vi "Initialize.vi"(8 "error in":errorcluster, 9 "Application Directory":path, 10 "Device":string, 11 "Oscilloscope in":refnum<class "Oscilloscope.lvclass">) -> (0 "error out":errorcluster, 3 "Oscilloscope out":refnum<class "Oscilloscope.lvclass">)   [LabVIEW 2019, in "Oscilloscope.lvlib" / "Oscilloscope.lvclass"]
uses:
  Oscilloscope.lvclass
  builds/Instruments/Instruments.lvlibp/Library/Instruments.lvclass
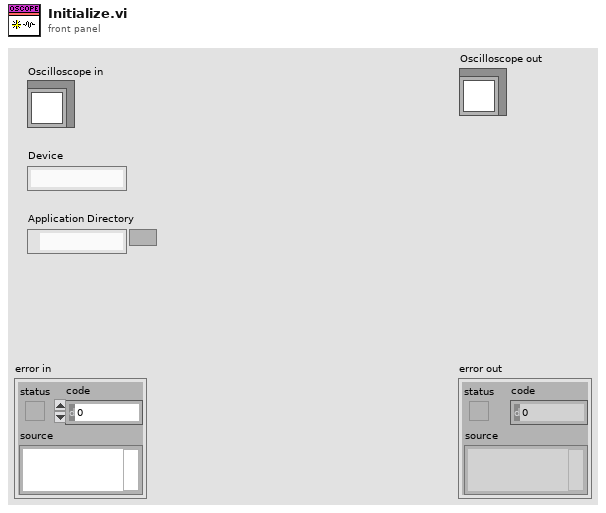
[diagram p1: front panel]
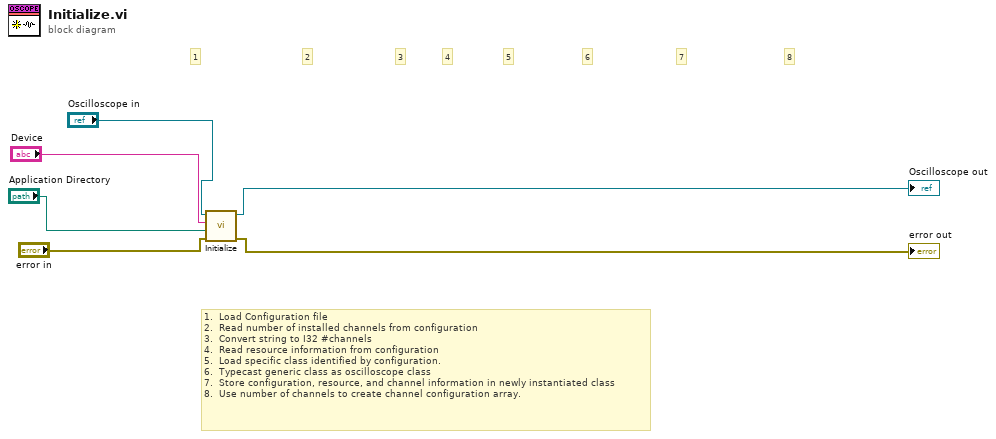
[diagram p0: block diagram]
diagram:
  # "1.  Load Configuration file\n2.  Read number of installed channels from configuration\n3.  Convert string to I32 #channels\n4.  Read resource information from configuration\n5.  Load specific class identified by configuration.\n6.  Typecast generic class as oscilloscope class\n7.  Store configuration, resource, and channel information in newly instantiated class\n8.  Use number of channels to create channel configuration array."
  # "8"
  # "7"
  # "6"
  # "5"
  # "4"
  # "3"
  # "2"
  # "1"
  n1 = call-parent "Initialize.vi"("error in"="error in", "Path"="Application Directory", "Device"="Device", "Instruments in"="Oscilloscope in") -> ("error out"=→"error out":errorcluster, "Instruments out"=→"Oscilloscope out":refnum<class "Oscilloscope.lvclass">)  [unwired: 6 in]
